vi "Inverse Filter Demo-2.vi"() -> ()   [LabVIEW 2015]
uses:
  Utility VIs/Math VIs/FFT x(t) to dB,Degrees (1D).vi
  Utility VIs/Math VIs/Linear to dB (array).vi
  Utility VIs/Math VIs/dB to Linear (1D).vi
panel:
  in  "T (s)":dbl
  in  "Fs (Hz)":dbl
  out "Noise out":cluster{"Frequency (Hz)":dbl[], "dB":dbl[]}[](graph)
  in  "Calibration file":path
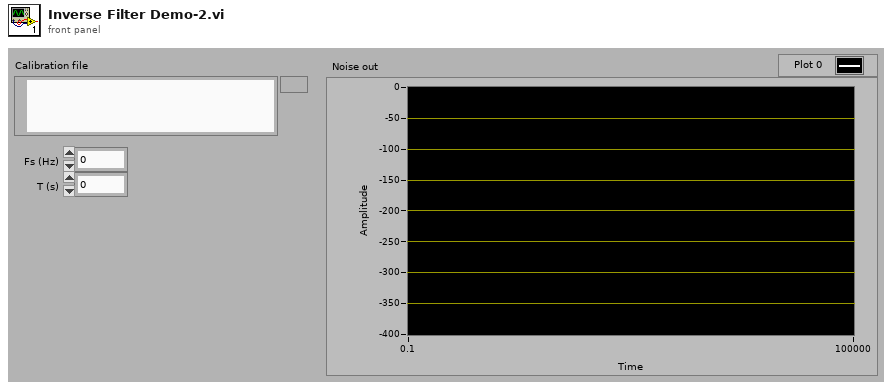
[diagram p1: front panel]
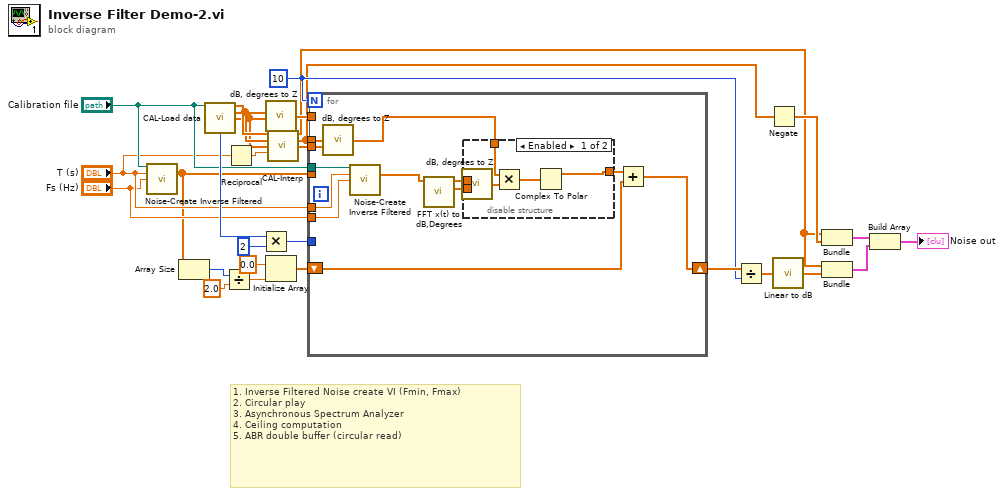
[diagram p0: block diagram]
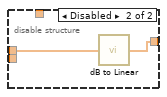
[diagram p2: hidden frame]
diagram:
  w21 = 10
  # "1. Inverse Filtered Noise create VI (Fmin, Fmax)\n2. Circular play\n3. Asynchronous Spectrum Analyzer\n4. Ceiling computation\n5. ABR double buffer (circular read)"
  n1 = call "Noise-Create Inverse Filtered.vi"("Calibration file"="Calibration file", "T (s)"="T (s)", "Fs (Hz)"="Fs (Hz)") -> ("Noise"=w6:dbl[])  [unwired: 11 in, 1 out]
  n2 = Array Size(array=w6) -> (size(s)=w7:i32)
  n3 = call "CAL-Load data.vi"("user path"="Calibration file") -> ("Frequency (Hz)"=w17:dbl[], "Mag"=w16:dbl[], "Phase"=w15:dbl[], "npts"=w23:i32)  [unwired: 7 in, 4 out]
  n4 = Divide(x=w7, y=2.0) -> (x/y=w9:dbl)
  n5 = Reciprocal(x="T (s)") -> (1/x=w13:dbl)
  n6 = Multiply(x=w23, y=2) -> (x*y=w27:i32)
  n7 = call "dB, degrees to Z.vi"("Magnitude (dB)"=w16, "Phase (degrees)"=w15) -> ("Z"=w28:cdb[])  [unwired: 5 in]
  n8 = Initialize Array(0.0 ("element"), w9) -> (w25:dbl[])
  n9 = call "CAL-Interp.vi"("Frequency (Hz)"=w17, "Magnitude (dB)"=w16, "Phase (degrees)"=w15, "df (Hz)"=w13) -> ("Interp Freq (Hz)"=w4:dbl[], "Interp Magnitude (dB)"=w3:dbl[], "Interp Phase (degrees)"=w14:dbl[])  [unwired: 8 in, 1 out]
  n10 = for {
    N: w21 -> [_]
    tunnel: w27 -> [_]
    tunnel: w28 -> [_]
    shift-right: [w39] -> w22
    shift-left: w25 -> [w38]
    tunnel: w6 -> [_]
    tunnel: w3 -> [w36]
    tunnel: w14 -> [w35]
    tunnel: "Calibration file" -> [w33]
    tunnel: "T (s)" -> [w32]
    tunnel: "Fs (Hz)" -> [w31]
    n11 = call "dB, degrees to Z.vi"("Magnitude (dB)"=w36, "Phase (degrees)"=w35) -> ("Z"=w34:cdb[])  [unwired: 5 in]
    n12 = call "Noise-Create Inverse Filtered.vi"("Calibration file"=w33, "T (s)"=w32, "Fs (Hz)"=w31) -> ("Noise"=w29:dbl[])  [unwired: 11 in, 1 out]
    n13 = call-poly "FFT x(t) to dB,Degrees.vi"("X"=w29) -> ("+Freq Phase of FFT (degrees)"=w40:dbl[], "+Freq. Mag of FFT (dB rms)"=w37:dbl[])  [unwired: 8 in, 1 out]
    n14 = disable-structure shown="Enabled" {
      disable-tunnel: w37 -> [w46 w48]
      disable-tunnel: w40 -> [w45 _]
      disable-tunnel: w34 -> [w43 _]
      disable-tunnel: [w41 w47] -> w30
      frame Enabled {
        n15 = call "dB, degrees to Z.vi"("Magnitude (dB)"=w46, "Phase (degrees)"=w45) -> ("Z"=w44:cdb[])  [unwired: 5 in]
        n16 = Multiply(x=w43, y=w44) -> (x*y=w42:cdb[])
        n17 = Complex To Polar(r * e^(i*theta)=w42) -> (r=w41:dbl[])  [unwired: 1 out]
      }
      frame Disabled {
        n18 = call-poly "dB to Linear.vi"("dB"=w48) -> ("linear"=w47:dbl[])
      }
    }
    n19 = Add(x=w30, y=w38) -> (x+y=w39:dbl[])
  }
  n20 = Divide(x=w22, y=w21) -> (x/y=w2:dbl[])
  n21 = Negate(x=w3) -> (-x=w18:dbl[])
  n22 = call-poly "Linear to dB.vi"("linear"=w2) -> ("dB"=w1:dbl[])
  n23 = Bundle("Interp Freq (Hz)"=w4, w18) -> (w5:cluster{"Interp Freq (Hz)":dbl[], dbl[]})  [unwired: 1 in]
  n24 = Bundle("Interp Freq (Hz)"=w4, "dB"=w1) -> (w20:cluster{"Interp Freq (Hz)":dbl[], "dB":dbl[]})  [unwired: 1 in]
  n25 = Build Array(w5, w20) -> (→"Noise out":cluster{"Interp Freq (Hz)":dbl[], "dB":dbl[]}[])
